vi "new.vi"(6 "stopTimeout[ms]":i32=5000, 8 "error in (no error)":errorcluster, 11 "task":refnum<class "ITask.lvclass">) -> (0 "error out":errorcluster, 3 "TaskController out":refnum<class "TaskController.lvclass">)   [LabVIEW 2023, in "TLC_Daemon.lvlib" / "TaskController.lvclass"]
doc: "Constructor\nNote: TaskController handles the life cycle of a single task.\nUse more TaskController objects if you want to handle more tasks."
uses:
  TaskController.lvclass
  ITask/ITask.lvclass
  status.ctl
  TaskController.lvclass/TaskController.ctl
  ITaskChannel/ITaskChannel.lvclass
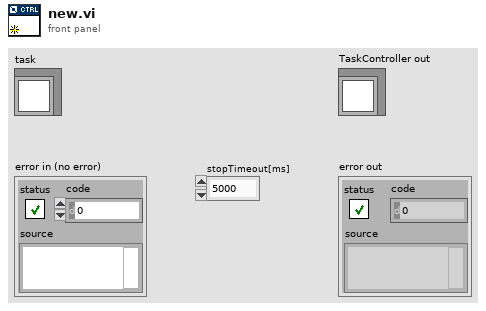
[diagram p1: front panel]
types:
  T1 = typedef "TLC_Daemon.lvlib/TaskController.lvclass/status.ctl" = enum16{"NotReady", "Ready", "Running", "Stopped", "Unknown"}
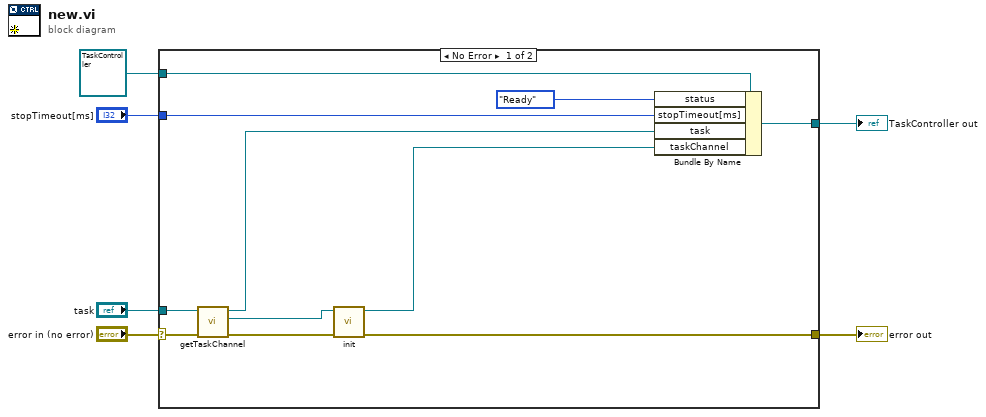
[diagram p0: block diagram]
diagram:
  n1 = case shown="No Error" "error in (no error)" {
    selector: "error in (no error)" -> [w15 w19]
    tunnel: [w9 w19] -> w5
    tunnel: [w16 w18] -> w3
    tunnel: refnum<class "TaskController.lvclass"> refnum ("TaskController in") -> [w17 w18]
    tunnel: "task" -> [w13 _]
    tunnel: "stopTimeout[ms]" -> [w7 _]
    frame No Error {
      n2 = call-dynamic "getTaskChannel.vi"("error in (no error)"=w15, "ITask in"=w13) -> ("error out"=w12:errorcluster, "stopMechanism"=w11:refnum<class "ITaskChannel.lvclass">, "ITask out"=w14:refnum<class "ITask.lvclass">)  [unwired: 7 in]
      n3 = call-dynamic "init.vi"("error in (no error)"=w12, "ITaskStopMechanism in"=w11) -> ("error out"=w9:errorcluster, "ITaskStopMechanism out"=w10:refnum<class "ITaskChannel.lvclass">)  [unwired: 8 in]
      n4 = Bundle By Name(cluster=w17, "status"=status."Ready", "stopTimeout[ms]"=w7, "task"=w14, "taskChannel"=w10) -> (w16:refnum<class "TaskController.lvclass">)
    }
    frame Error {
    }
  }
  "error out" <- w5
  "TaskController out" <- w3
